vi "Tare-To_Dynamic.vi"(9 "Tare In":bool, 11 "Waveform":waveform(dbl)) -> (3 "Dynamic Data Type":dynamicdata(waveform))   [LabVIEW 2025]
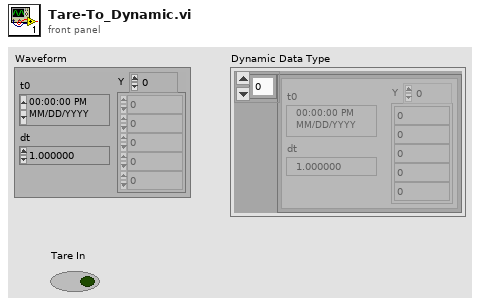
[diagram p1: front panel]
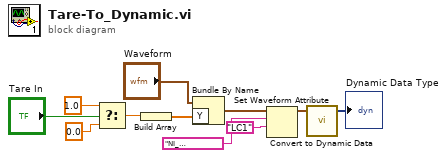
[diagram p0: block diagram]
diagram:
  n1 = Select(t=1.0, s="Tare In", f=0.0) -> (s? t:f=w4:dbl)
  n2 = Build Array(w4) -> (w5:dbl[])
  n3 = Bundle By Name(cluster="Waveform", "Y"=w5) -> (w11:waveform(dbl))
  n4 = Set Waveform Attribute(5:"LC1" ("name"), 6:"NI_ChannelName" ("name"), 7:w11) -> (3:w8:waveform(dbl))  [unwired: 1 in, 2 out]
  n5 = call "Convert to Dynamic Data"("Waveform"=w8) -> ("Dynamic Data Type"=→"Dynamic Data Type":dynamicdata)  [unwired: 3 in]
